vi "Programme Élémentaire VI_Tree.vi"   [LabVIEW 2020]
doc: "This is the instrument driver for the <B> elc ALR 3220 </B> Power Supply.. \nThe VI Tree displays all the user-callable VIs of the instrument driver in an organized table."
panel:
  # "(c) 2005-2018 National Instruments.  ALL RIGHTS RESERVED."
  # "© 2008-2020 elc  CORPORATION ALL RIGHTS RESERVED."
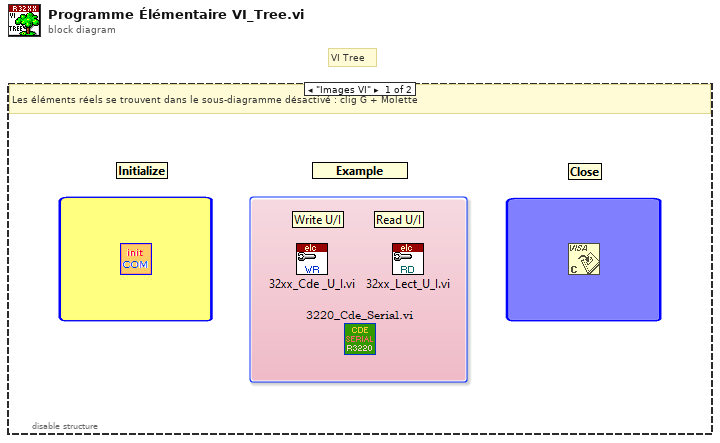
[diagram p0: block diagram]
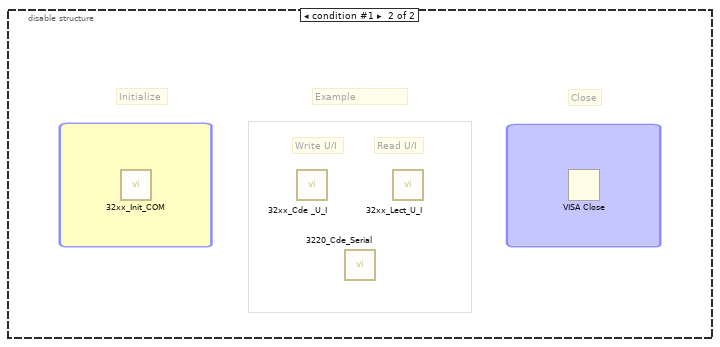
[diagram p2: hidden frame]
diagram:
  # "VI Tree"
  n1 = disable-structure shown="\"Images VI\"" {
    frame condition #0 (active) {
      # "Les éléments réels se trouvent dans le sous-diagramme désactivé : clig G + Molette"
    }
    frame condition #1 {
      # "Read U/I"
      # "Write U/I"
      # "Example"
      # "Close"
      # "Initialize"
      n2 = call "32xx_Init_COM.vi"() -> ()  [unwired: 9 in, 3 out]
      n3 = call "32xx_Cde _U_I.vi"() -> ()  [unwired: 10 in, 2 out]
      n4 = call "3220_Cde_Serial.vi"() -> ()  [unwired: 8 in, 4 out]
      n5 = call "32xx_Lect_U_I.vi"() -> ()  [unwired: 10 in, 2 out]
      n6 = VISA Close() -> ()  [unwired: 2 in, 1 out]
    }
  }
